vi "CreatePrivateEvents.vi"(8 "error in (no error)":errorcluster, 11 "demoForJoe":refnum<class "demoForJoe.lvclass">) -> (0 "error out":errorcluster, 3 "demoForJoe out":refnum<class "demoForJoe.lvclass">)   [LabVIEW 2016, in "demoForJoe.lvclass"]
doc: "---------------------------------------------------------------\nJKI State Machine Objects™\nhttp://jki.net/state-machine-objects/\nCopyright (C) 2005-2015, JKI <info@jki.net>\nALL RIGHTS RESERVEDJKI State Machine Objects (SMO) 1.0.0.4\nJKI - JKI\nCopyright (c) 2015, JKI"
uses:
  demoForJoe.lvclass
  Typedefs/PrivateEvents--demoForJoe.StringMethod.ctl
  demoForJoe.lvclass/demoForJoe.ctl
  <vilib>/JKI/JKI SMO/SMO/SMO.lvclass
panel:
  # "For instructions on how to use the JKI State Machine Objects, examples and video tutorials, visit:\nhttp://jki.net/state-machine-objects/\n\nJKI State Machine Objects™\nhttp://jki.net/state-machine-objects/\nCopyright (C) 2005-2015, JKI <info@jki.net>\nALL RIGHTS RESERVED"
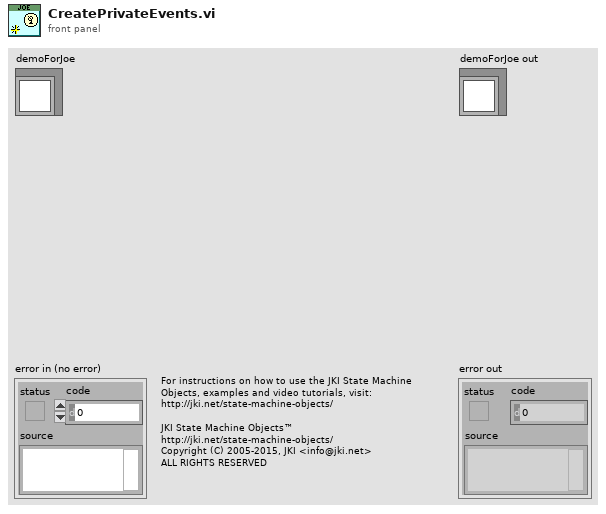
[diagram p1: front panel]
types:
  T1 = typedef "demoForJoe.lvclass/PrivateEvents--demoForJoe.StringMethod.ctl" = string
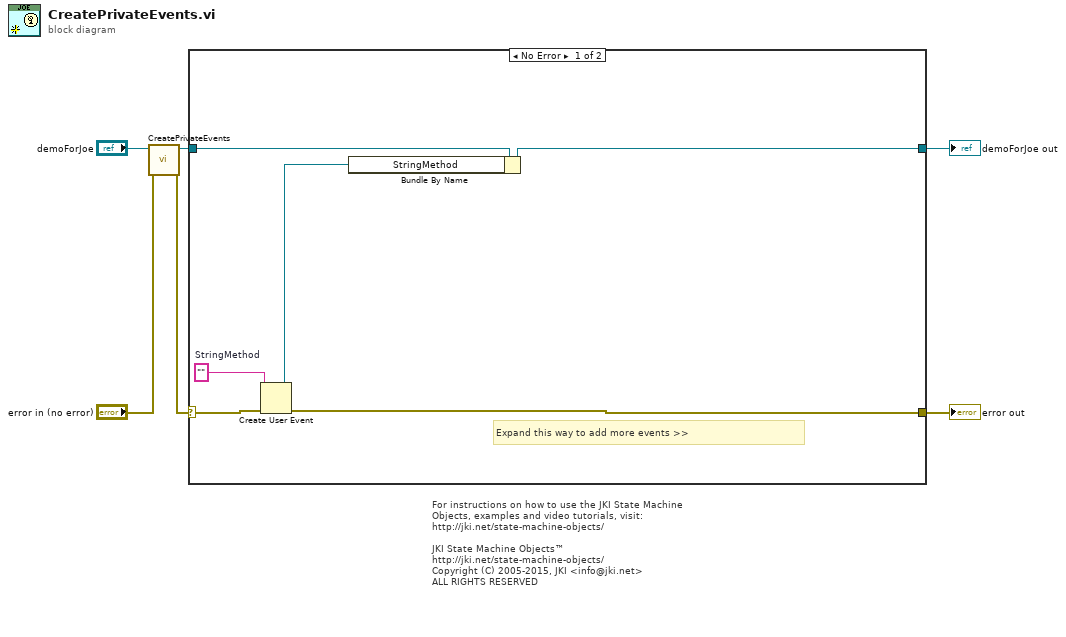
[diagram p0: block diagram]
diagram:
  # "For instructions on how to use the JKI State Machine Objects, examples and video tutorials, visit:\nhttp://jki.net/state-machine-objects/\n\nJKI State Machine Objects™\nhttp://jki.net/state-machine-objects/\nCopyright (C) 2005-2015, JKI <info@jki.net>\nALL RIGHTS RESERVED"
  n1 = call-parent "CreatePrivateEvents.vi"("error in (no error)"="error in (no error)", "SMO"="demoForJoe") -> ("error out"=w1:errorcluster, "SMO out"=w3:refnum<class "demoForJoe.lvclass">)  [unwired: 8 in]
  n2 = case shown="No Error" w1 {
    selector: w1 -> [w11 w14]
    tunnel: [w9 w14] -> w5
    tunnel: [w10 w13] -> w6
    tunnel: w3 -> [w12 w13]
    frame No Error {
      w8 = T1 ""  # StringMethod
      # "Expand this way to add more events >>"
      n3 = Create User Event(user event datatype=w8, error in=w11) -> (user event=w7:refnum<user-event>, error out=w9:errorcluster)
      n4 = Bundle By Name(cluster=w12, "StringMethod"=w7) -> (w10:refnum<class "demoForJoe.lvclass">)
    }
    frame Error {
    }
  }
  "error out" <- w5
  "demoForJoe out" <- w6
